vi "Turn.vi"(10 "Angle":dbl, 11 "Effort":dbl) -> ()   [LabVIEW 2016]
uses:
  <vilib>/Rock Robotics/WPI/SafetyOutput/WPI_SafetyOutputConfigMenu.ctl
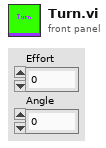
[diagram p1: front panel]
types:
  T1 = typedef "WPI_SafetyOutputConfigMenu.ctl" = enum16{"Enable", "Disable"}
  T2 = typedef "WPI_GyroDevRef.ctl" = cluster{"DevStatus":errorcluster, "Analog Channel":T3, "Offset":dbl, "Gain (VoltsPerDegree/Second)":dbl, "Gyro Type":enum16{"Analog", "XRS450"}, "Handle":i32, "SPI Bus":T4, "Device Found":bool, "Sample Rate":dbl, "Calibrate On Open":bool}
  T3 = typedef "FPGA_AIChannel.ctl" = enum8{"AI 0", "AI 1", "AI 2", "AI 3", "AI MXP 0", "AI MXP 1", "AI MXP 2", "AI MXP 3", "Invalid"}
  T4 = typedef "spi_bus.ctl" = enum16{"SPI On-Board, CS0", "SPI On-Board, CS1", "SPI On-Board, CS2", "SPI On-Board, CS3", "SPI MXP", "Invalid"}
  T5 = typedef "WPI_MotorControlDeviceRef.ctl" = cluster{"DeviceStatus":errorcluster, "Type":T6, "PWM":cluster{"PWM Channel":T7, "DeadBand":T8}, "CAN":cluster{"Device Number":u8, "SetOutput VI Ref":variant, "GetOutput VI Ref":variant, "Enable VI Ref":variant, "Disable VI Ref":variant, "Data":variant}, "Invert":bool}
  T6 = typedef "WPI_MotorControlType.ctl" = enum16{"PWM", "CAN"}
  T7 = typedef "FPGA_DIOPWMChannel.ctl" = enum8{"PWM 0", "PWM 1", "PWM 2", "PWM 3", "PWM 4", "PWM 5", "PWM 6", "PWM 7", "PWM 8", "PWM 9", "PWM MXP 0", "PWM MXP 1", "PWM MXP 2", "PWM MXP 3", "PWM MXP 4", "PWM MXP 5", "PWM MXP 6", "PWM MXP 7", "PWM MXP 8", "PWM MXP 9", "Invalid"}
  T8 = typedef "WPI_PWMDeadband.ctl" = cluster{"Name":string, "maxPositivePwm":i32, "minPositivePwm":i32, "centerPwm":i32, "maxNegativePwm":i32, "minNegativePwm":i32, "angularRange":u16}
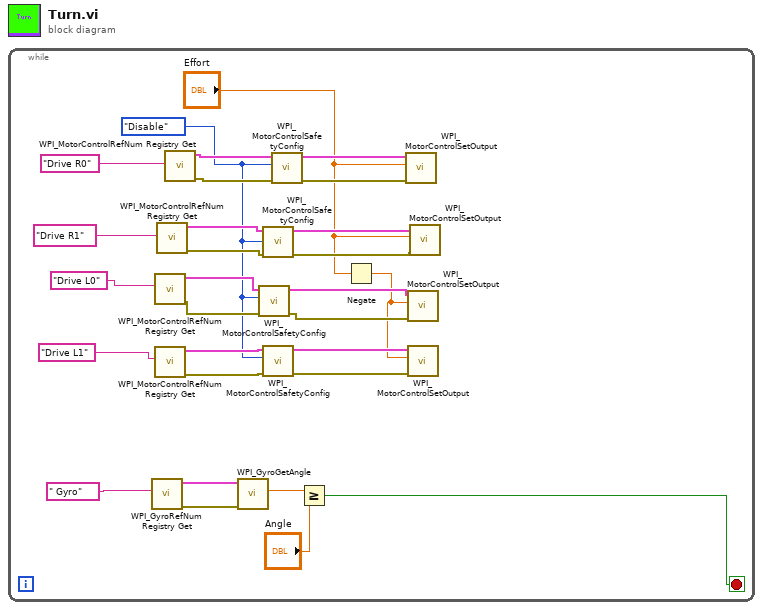
[diagram p0: block diagram]
diagram:
  n1 = while {
    stop <- w7 stop-if-true
    w14 = WPI_SafetyOutputConfigMenu."Disable" ("mode")
    n2 = call <vilib>:"WPI_GyroRefNum Registry Get.vi"("refnum name"=" Gyro") -> ("error out"=w9:errorcluster, "GyroDevRef"=w10:T2)  [unwired: 9 in]
    n3 = call <vilib>:"WPI_MotorControlRefNum Registry Get.vi"("refnum name"="Drive L0") -> ("error out"=w19:errorcluster, "MotorControlDevRef"=w24:T5)  [unwired: 9 in]
    n4 = call <vilib>:"WPI_MotorControlRefNum Registry Get.vi"("refnum name"="Drive L1") -> ("error out"=w18:errorcluster, "MotorControlDevRef"=w22:T5)  [unwired: 9 in]
    n5 = call <vilib>:"WPI_MotorControlRefNum Registry Get.vi"("refnum name"="Drive R1") -> ("error out"=w25:errorcluster, "MotorControlDevRef"=w27:T5)  [unwired: 9 in]
    n6 = call <vilib>:"WPI_MotorControlRefNum Registry Get.vi"("refnum name"="Drive R0") -> ("error out"=w28:errorcluster, "MotorControlDevRef"=w29:T5)  [unwired: 9 in]
    n7 = call <vilib>:"WPI_GyroGetAngle.vi"("error in"=w9, "GyroDevRef"=w10) -> ("Angle"=w8:dbl)  [unwired: 5 in, 4 out]
    n8 = call <vilib>:"WPI_MotorControlSafetyConfig.vi"("error in (no error)"=w19, "mode"=w14, "MotorControlDevRef"=w24) -> ("error out"=w20:errorcluster, "MotorControlDevRef"=w23:T5)  [unwired: 7 in]
    n9 = call <vilib>:"WPI_MotorControlSafetyConfig.vi"("error in (no error)"=w25, "mode"=w14, "MotorControlDevRef"=w27) -> ("error out"=w13:errorcluster, "MotorControlDevRef"=w26:T5)  [unwired: 7 in]
    n10 = call <vilib>:"WPI_MotorControlSafetyConfig.vi"("error in (no error)"=w18, "mode"=w14, "MotorControlDevRef"=w22) -> ("error out"=w17:errorcluster, "MotorControlDevRef"=w21:T5)  [unwired: 7 in]
    n11 = call <vilib>:"WPI_MotorControlSafetyConfig.vi"("error in (no error)"=w28, "mode"=w14, "MotorControlDevRef"=w29) -> ("error out"=w12:errorcluster, "MotorControlDevRef"=w16:T5)  [unwired: 7 in]
    n12 = Greater Or Equal?(x=w8, y="Angle") -> (x >= y?=w7:bool)
    n13 = Negate(x="Effort") -> (-x=w15:dbl)
    n14 = call <vilib>:"WPI_MotorControlSetOutput.vi"("error in (no error)"=w12, "Output"="Effort", "MotorControlDevRef"=w16) -> ()  [unwired: 6 in, 3 out]
    n15 = call <vilib>:"WPI_MotorControlSetOutput.vi"("error in (no error)"=w20, "Output"=w15, "MotorControlDevRef"=w23) -> ()  [unwired: 6 in, 3 out]
    n16 = call <vilib>:"WPI_MotorControlSetOutput.vi"("error in (no error)"=w17, "Output"=w15, "MotorControlDevRef"=w21) -> ()  [unwired: 6 in, 3 out]
    n17 = call <vilib>:"WPI_MotorControlSetOutput.vi"("error in (no error)"=w13, "Output"="Effort", "MotorControlDevRef"=w26) -> ()  [unwired: 6 in, 3 out]
  }
